vi "cal.vi"() -> ()   [LabVIEW 2014]
panel:
  out "Numeric 3":dbl
  in  "Numeric 2":dbl
  in  "Numeric":dbl
  in  "Enum":T1(ring)
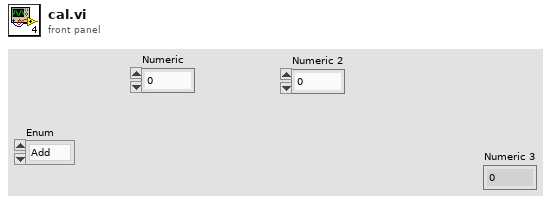
[diagram p1: front panel]
types:
  T1 = enum16{"Add", "Sub", "Mul", "Div", "Sq", "Sq root", "Avg", "Max", "Min"}
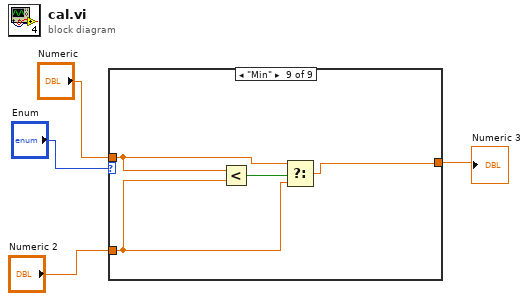
[diagram p0: block diagram]
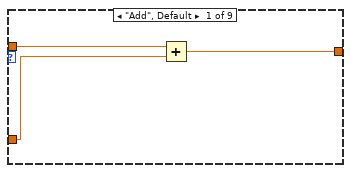
[diagram p2: hidden frame]
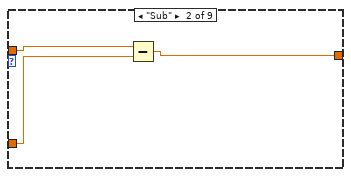
[diagram p3: hidden frame]
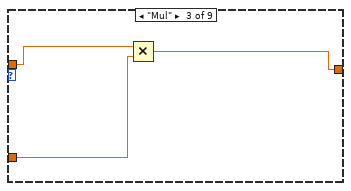
[diagram p4: hidden frame]
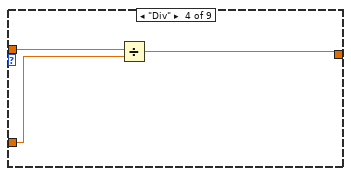
[diagram p5: hidden frame]
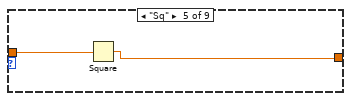
[diagram p6: hidden frame]
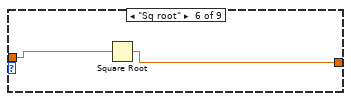
[diagram p7: hidden frame]
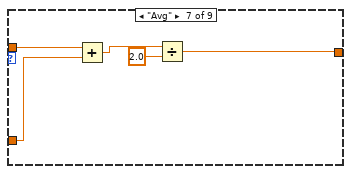
[diagram p8: hidden frame]
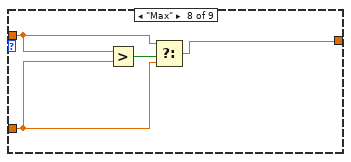
[diagram p9: hidden frame]
diagram:
  n1 = case shown="\"Min\"" "Enum" {
    tunnel: "Numeric" -> [w7 w10 w13 w16 w18 w20 w25 w27 w32]
    tunnel: "Numeric 2" -> [w6 w9 w12 w15 _ _ w24 w28 w31]
    tunnel: [w5 w8 w11 w14 w17 w19 w21 w26 w30] -> w1
    frame "Add", Default {
      n2 = Add(x=w7, y=w6) -> (x+y=w5:dbl)
    }
    frame "Sub" {
      n3 = Subtract(x=w10, y=w9) -> (x-y=w8:dbl)
    }
    frame "Mul" {
      n4 = Multiply(x=w13, y=w12) -> (x*y=w11:dbl)
    }
    frame "Div" {
      n5 = Divide(x=w16, y=w15) -> (x/y=w14:dbl)
    }
    frame "Sq" {
      n6 = Square(x=w18) -> (x^2=w17:dbl)
    }
    frame "Sq root" {
      n7 = Square Root(x=w20) -> (sqrt(x)=w19:dbl)
    }
    frame "Avg" {
      n8 = Add(x=w25, y=w24) -> (x+y=w23:dbl)
      n9 = Divide(x=w23, y=2.0) -> (x/y=w21:dbl)
    }
    frame "Max" {
      n10 = Greater?(x=w27, y=w28) -> (0:w29:bool)
      n11 = Select(t=w27, s=w29, f=w28) -> (s? t:f=w26:dbl)
    }
    frame "Min" {
      n12 = Less?(x=w32, y=w31) -> (x < y?=w33:bool)
      n13 = Select(t=w32, s=w33, f=w31) -> (s? t:f=w30:dbl)
    }
  }
  "Numeric 3" <- w1
